vi "单个流程写入.vi"(5 "简易流程Id":u16(ring), 6 "是否是简易流程":bool, 7 "添加的路径":path, 8 "error in (no error)":errorcluster caption="错误输入（无错误）", 9 "量程":enum16{"低量程", "高量程"}(ring), 10 "测量模式":T1(ring), 11 "测量参数":u16(ring) items=["总氮"=2, "总磷"=1, "氨氮"=3, "COD"=22]) -> (0 "error out":errorcluster caption="错误输出", 2 "交织的数组":u16[](array[numeric]) format="0x%04x", 3 "步数":i32)   [LabVIEW 2016, in "斯坦道氟化物.lvlib"]
panel:
  out "大小 2":i32
  out "流程写入进度":dbl
  out "大小":i32
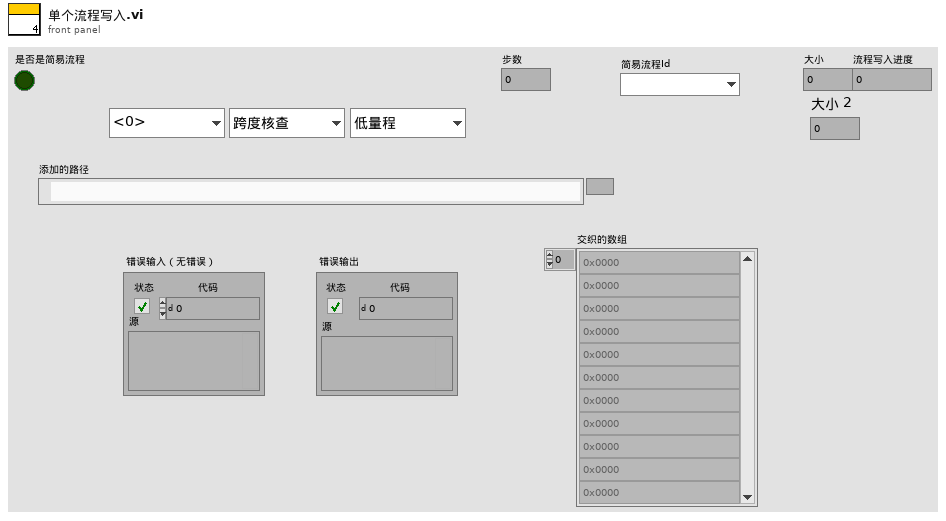
[diagram p1: front panel]
types:
  T1 = enum16{"跨度核查", "水样测量", "零点核查", "标样核查", "加标回收", "快捷测试", "空白校准", "标样校准"}
  T2 = cluster{"测量参数":u16, "测量模式":enum16{"跨度核查", "水样测量", "零点核查", "标样核查", "加标回收", "快捷测试", "空白校准", "标样校准"}, "量程":enum16{"低量程", "高量程"}}
  T3 = cluster{"port":i32, "dac":u8, "adc":u8, "time":u16, "步骤名":string}[]
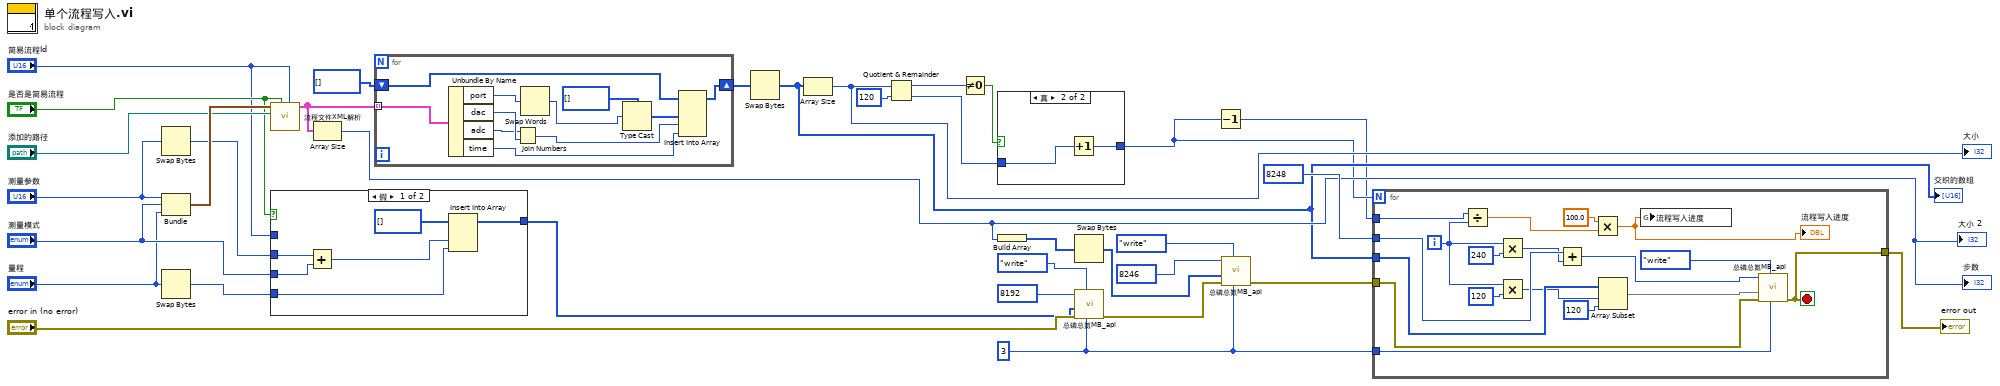
[diagram p0: block diagram]
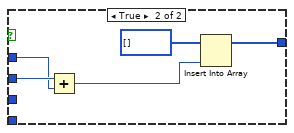
[diagram p3: hidden frame]
diagram:
  w8 = 3
  n1 = Swap Bytes(anything="测量参数") -> (byte swapped=w16:u16)
  n2 = Bundle("测量参数"="测量参数", "测量模式"="测量模式", "量程"="量程") -> (w24:T2)  [unwired: 1 in]
  n3 = Swap Bytes(anything="量程") -> (byte swapped=w11:u16)
  n4 = call "流程文件XML解析.vi"("简易流程Id"="简易流程Id", "是否是简易流程"="是否是简易流程", "添加的路径"="添加的路径", "参数簇"=w24) -> ("数组"=w20:T3)  [unwired: 7 in]
  n5 = case shown="假" "是否是简易流程" {
    tunnel: [w38 w43] -> w28
    tunnel: "测量模式" -> [w37 _]
    tunnel: w16 -> [w36 w42]
    tunnel: w11 -> [w35 _]
    tunnel: "简易流程Id" -> [_ w41]
    frame False {
      n6 = Add(x=w36, y=w37) -> (x+y=w40:u16)
      n7 = Insert Into Array(array=u16[] [] ("数组"), new element #1=w40, new element #2=w35) -> (w38:u16[])  [unwired: 1 in]
    }
    frame True {
      n8 = Add(x=w42, y=w41) -> (x+y=w45:u16)
      n9 = Insert Into Array(array=u16[] [] ("数组"), new element=w45) -> (w43:u16[])  [unwired: 1 in]
    }
  }
  n10 = Array Size(array=w20) -> (size(s)=w17:i32)
  "步数" <- w17
  "大小 2" <- w17
  n11 = for {
    tunnel: w20 -> [w56] mode=indexing
    shift-right: [w51] -> w21
    shift-left: u16[] [] -> [w49]
    n12 = Unbundle By Name(w56) -> ("port"=w54:i32, "dac"=w47:u8, "adc"=w46:u8, "time"=w52:u16)
    n13 = Join Numbers(hi=w46, lo=w47) -> ((hi.lo)=w53:u16)
    n14 = Swap Words(1:w54) -> (0:w48:i32)
    n15 = Type Cast(type=u16[] [], x=w48) -> (*(type *) &x=w50:u16[])
    n16 = Insert Into Array(array=w49, new element #1=w50, new element #2=w53, new element #3=w52) -> (w51:u16[])  [unwired: 1 in]
  }
  n17 = Swap Bytes(anything=w21) -> (byte swapped=w9:u16[])
  "交织的数组" <- w9
  n18 = Array Size(array=w9) -> (size(s)=w7:i32)
  "大小" <- w7
  n19 = Quotient & Remainder(x=w7, y=120) -> (x-y*floor(x/y)=w5:i32, floor(x/y)=w3:i32)
  n20 = Not Equal To 0?(x=w5) -> (x != 0?=w4:bool)
  n21 = case shown="真" w4 {
    tunnel: w3 -> [w57 w59]
    tunnel: [w57 w58] -> w2
    frame False {
    }
    frame True {
      n22 = Increment(x=w59) -> (x+1=w58:i32)
    }
  }
  n23 = Build Array(w17) -> (w19:i32[])
  n24 = Swap Bytes(anything=w19) -> (byte swapped=w18:i32[])
  n25 = call "总磷总氮MB_api.vi"("Slave ID"=w8, "STEP"=enum16{"open", "read", "write", "close"}."write", "Error in"="error in (no error)", "values"=w28, "starting address"=u16 8192) -> ("error out"=w31:errorcluster)  [unwired: 4 in, 2 out]
  n26 = Decrement(x=w2) -> (x-1=w1:i32)
  n27 = call "总磷总氮MB_api.vi"("Slave ID"=w8, "STEP"=enum16{"open", "read", "write", "close"}."write", "Error in"=w31, "values"=w18, "starting address"=u16 8246) -> ("error out"=w27:errorcluster)  [unwired: 4 in, 2 out]
  n28 = for {
    N: w2 -> [_]
    tunnel: u16 8248 ("starting address") -> [w73]
    tunnel: w27 -> [w77]
    tunnel: [w75] -> w25
    tunnel: w9 -> [w67]
    tunnel: w8 -> [w62]
    tunnel: w1 -> [w60]
    i -> [w65]
    stop <- w75 stop-if-true
    n29 = Divide(x=w60, y=w65) -> (x/y=w70:dbl)
    n30 = Multiply(x=w65, y=240) -> (x*y=w72:i32)
    n31 = Multiply(x=w65, y=120) -> (x*y=w64:i32)
    n32 = Add(x=w73, y=w72) -> (x+y=w74:i32)
    n33 = Multiply(x=100.0, y=w70) -> (x*y=w68:dbl)
    "流程写入进度" <- w68
    n34 = Array Subset(array=w67, index=w64, length=120 ("长度")) -> (w63:u16[])
    n35 = global write "VAR总磷总氮全局变量.vi" "流程写入进度"(w68) -> ()
    n36 = call "总磷总氮MB_api.vi"("Slave ID"=w62, "STEP"=enum16{"open", "read", "write", "close"}."write", "Error in"=w77, "values"=w63, "starting address"=w74) -> ("error out"=w75:errorcluster)  [unwired: 4 in, 2 out]
  }
  "error out" <- w25
